vi "TECATCal.vi"(10 "dZeroLvl":dbl=2.544 format="%.3g", 11 "wfmIN":waveform(dbl)) -> (3 "wfmOUT":waveform(dbl))   [LabVIEW 2017]
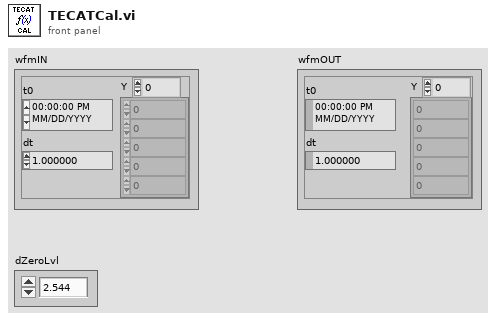
[diagram p1: front panel]
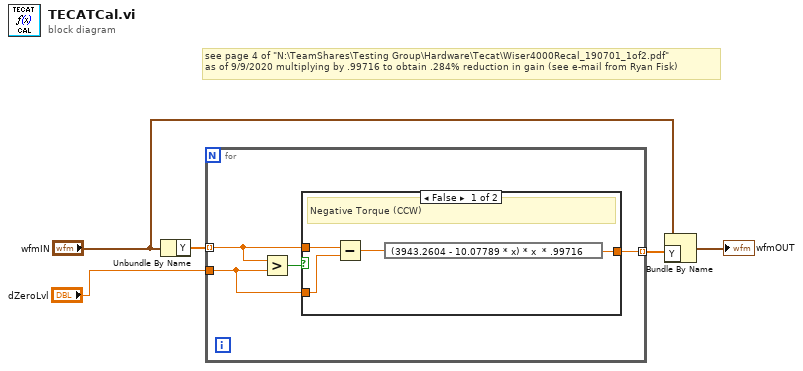
[diagram p0: block diagram]
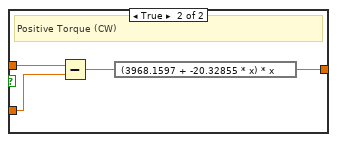
[diagram p2: hidden frame]
diagram:
  # "see page 4 of \"N:\\TeamShares\\Testing Group\\Hardware\\Tecat\\Wiser4000Recal_190701_1of2.pdf\"\nas of 9/9/2020 multiplying by .99716 to obtain .284% reduction in gain (see e-mail from Ryan Fisk)"
  n1 = Unbundle By Name("wfmIN") -> ("Y"=w5:dbl[])
  n2 = for {
    tunnel: w5 -> [w8] mode=indexing
    tunnel: "dZeroLvl" -> [w6]
    tunnel: [w7] -> w2 mode=indexing
    n3 = Greater?(x=w8, y=w6) -> (0:w9:bool)
    n4 = case shown="False" w9 {
      tunnel: w8 -> [w12 w16]
      tunnel: [w13 w17] -> w7
      tunnel: w6 -> [w11 w15]
      frame False {
        # "Negative Torque (CCW)"
        n5 = Subtract(x=w12, y=w11) -> (x-y=w10:dbl)
        n6 = expression code="(3943.2604 - 10.07789 * x) * x  * .99716"(w10) -> (w13:dbl)
      }
      frame True {
        # "Positive Torque (CW)"
        n7 = Subtract(x=w16, y=w15) -> (x-y=w14:dbl)
        n8 = expression code="(3968.1597 + -20.32855 * x) * x"(w14) -> (w17:dbl)
      }
    }
  }
  n9 = Bundle By Name(cluster="wfmIN", "Y"=w2) -> (→"wfmOUT":waveform(dbl))
